vi "Dashboard Main.vi"() -> ()   [LabVIEW 2016]
uses:
  <vilib>/Utility/miscctls.llb/LVRowAndColumnTypeDef.ctl
  <vilib>/event_ctls.llb/eventvkey.ctl
  <vilib>/Rock Robotics/Network Tables/NT Read Numeric Array.vi
  <vilib>/Rock Robotics/Network Tables/NT Write Boolean.vi
  <vilib>/Rock Robotics/Network Tables/NT Read Boolean.vi
  <vilib>/Rock Robotics/WPI/Dashboard/WPI_DashboardLogging Global.vi
panel:
  in  "Camera Settings Right":T1={"Frame Rate"=30, "Compression"=30, "Size"=1, "DB Camera Config"=FALSE} {"Frame Rate" scale=1.0..30.0; "Compression" scale=100.0..-1.0; "Size" items=["640x480", "320x240", "160x120"]}
  in  "Camera Name Right":string(combo)="No Camera Selection"
  out "Camera Info":cluster{"Mbps LED":bool, "Mbps":dbl, "fps":dbl} {"fps" format="%#.1g"; "Mbps" format="%#.1g"}
  in  "Camera Settings":T1={"Frame Rate"=30, "Compression"=30, "Size"=1, "DB Camera Config"=FALSE} {"Frame Rate" scale=1.0..30.0; "Compression" scale=100.0..-1.0; "Size" items=["640x480", "320x240", "160x120"]}
  in  "TCP":refnum<k5>
  in  "Rec Mode":enum32{"Stop", "Record", "Playback"}(radio)
  out "Robot IP":string
  out "Image Message":string="Timeout in Camera Communications"
  in  "Dashboard Tab":T2(tab)
  out "Auto Aim":bool
  out "Vision Degrees":dbl
  out "Distance":dbl
  out "Score":dbl
  out "Shooter":bool
  in  "Compressor":bool
  in  "Delay":dbl(slide) scale=0.0..10.0
  out "RPM":dbl(knob) scale=0.0..10.0
  out "Right":dbl
  out "Left":dbl
  in  "Select Auto":string(combo)="Select Autonomous ..."
  out "NT Connection":bool
  out "MotorChart R":cluster{"Numeric":dbl, "Numeric":dbl}(graph)
  out "MotorChart L":cluster{"Numeric":dbl, "Numeric":dbl}(graph)
  out "MotorSliders R":cluster{"MotorSlide1":dbl, "MotorSlide2":dbl} {"MotorSlide2" scale=-1.0..1.0 scale format="%#_2e"; "MotorSlide1" scale=-1.0..1.0 scale format="%#_2e"}
  out "MotorSliders L":cluster{"MotorSlide1":dbl, "MotorSlide2":dbl} {"MotorSlide2" scale=-1.0..1.0 scale format="%#_2e"; "MotorSlide1" scale=-1.0..1.0 scale format="%#_2e"}
  out "Gyro":dbl(knob) scale=0.0..360.0
  out "JS1 Z":dbl(slide) scale=-1.0..1.0 scale format="%#_2e"
  out "JS1 Graph":cluster{"X":dbl, "Y":dbl}[](graph)
  out "JS1 Buttons":T3
  out "JS2 Z":dbl(slide) scale=-1.0..1.0 scale format="%#_2e"
  out "JS2 Graph":cluster{"X":dbl, "Y":dbl}[](graph)
  out "JS2 Buttons":T3
  out "Mode":T4(ring)=enum."Auto Disabled"
  out "Camera Image Right":T5(plugin-control)
  in  "DB/String 9":string
  in  "DB/String 8":string
  in  "DB/String 7":string
  in  "DB/String 6":string
  in  "DB/String 5":string
  in  "DB/String 4":string
  in  "DB/String 3":string
  in  "DB/String 2":string
  in  "DB/String 1":string
  in  "DB/String 0":string
  in  "DB/Slider 0":dbl(slide) scale=0.0..5.0
  in  "DB/Slider 1":dbl(slide) scale=0.0..5.0
  in  "DB/Slider 2":dbl(slide) scale=0.0..5.0
  in  "DB/Slider 3":dbl(slide) scale=0.0..5.0
  out "DB/LED 3":bool
  out "DB/LED 2":bool
  out "DB/LED 1":bool
  out "DB/LED 0":bool
  in  "DB/Button 3":bool
  in  "DB/Button 2":bool
  in  "DB/Button 1":bool
  in  "DB/Button 0":bool caption="New Name"
  in  "Test Slider":dbl(slide) scale=0.0..100.0 scale format="%#_3g"
  in  "On/Off":bool caption="Solenoid"
  in  "Test Name":u16(ring) items=["Select the test to run..."]
  in  "Test Tree":string(tree)
  in  "Motor":cluster{"Value":dbl, "Enable":bool} {"Value" scale=-1.0..1.0 scale format="%#_3g"}
  out "Progress":T6 {"Test Progress" scale=0.0..100.0}
  in  "Rev/Fwd":cluster{"Forward":bool, "Reverse":bool}
  in  "Test Ring":u16(ring) items=["Monochrome", "Color"]
  out "Cmd Status":string
  in  "Execute Command":bool
  in  "Command Params":string[][](table)
  in  "Command Selection":i32(listbox)
  in  "CheckList":i32(listbox)
  out "Tree":string(tree)
  out "Camera Image":T5(plugin-control)
  out "Background":bool
  in  "Camera Name":string(combo)="No Camera Selection"
  # "HW"
  # "HW"
  # "Joysticks"
  # "Drive Motors"
  # "Front"
  # "Right"
  # "Left"
  # "Back"
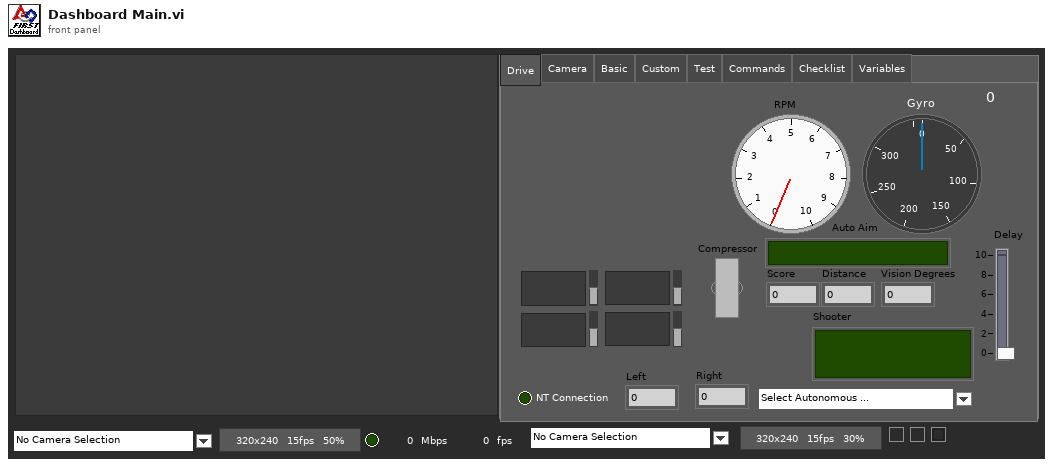
[diagram p1: front panel]
types:
  T1 = cluster{"Frame Rate":i32, "Compression":i32, "Size":u16, "DB Camera Config":bool}
  T2 = enum32{"Drive", "Camera", "Basic", "Custom", "Test", "Commands", "Checklist", "Variables"}
  T3 = cluster{bool, bool, bool, bool, bool, bool, bool, bool, bool, bool, bool, bool}
  T4 = enum8{"Tele-Op Disabled", "Tele-Op Enabled", "Auto Disabled", "Auto Enabled", "Test Disabled", "Test Enabled", "Disconnected", "No Code", "E-Stop"}
  T5 = typedef "IMAQ Image.ctl" = refnum<image>
  T6 = cluster{"Test Progress":u8, "Test Progress Text":string}
  T7 = typedef "Image Type" = u32
  T8 = cluster{"IDs":cluster{"RPC field ID":u16, "Unique ID":u16}, "String":string}
  T9 = enum32{"Drive", "Basic", "Custom", "Test", "Checklist", "Variables"}
  T10 = cluster{"Error Strings":string, "Disable Counts":cluster{u16, u16}, "Rail Faults":cluster{u16, u16, u16}, "Robot IP":string, "DB Mode":u8, "Event Info":cluster{"Name":string, "Type":u8, "Number":u16, "Replay":u8}}
  T11 = cluster{"Storage":cluster{"Disk Free":u64, "RAM Block":u32, "RAM free":u32}, "CPU Utilization":cluster{"CPU % ISR":sgl, "CPU % Time Crit":sgl, "CPU % Timed Str":sgl, "CPU % High":sgl, "CPU % Above":sgl, "CPU % Normal":sgl, "CPU % Low":sgl}, "CAN":cluster{"% Bus Utilization":sgl, "Bus Off Cnt":u32, "TX_FIFO Full Cnt":u32, "Receive Error Cnt":u8, "Transmit Error Cnt":u8}, "HID":cluster{"HID Outputs":u32, "Rumble Low":u16, "Rumble High":u16}[]}
  T12 = cluster{"Status bits":cluster{"Test Mode":bool, "Autonomous":bool, "Enabled":bool, "Code Start":bool, "Brownout":bool, "Reserved 2":bool, "Reserved 3":bool, "E-Stop":bool}, "Code Trace":cluster{"Disabled":bool, "TeleOp":bool, "Auto":bool, "Test":bool}, "Controller Type":enum16{"unknown", "cRIO", "roboRio"}, "Code?":enum16{"unknown", "noCode", "code"}, "Battery V":dbl}
  T13 = cluster{"Control Bits":cluster{"TestMode":bool, "Autonomous":bool, "Enabled":bool, "FMS Present":bool, bool, bool, bool, "E-Stop":bool}, "Team Station ":u8, "Countdown":sgl, "Joystick Values":cluster{"Axes":dbl[], "Buttons":bool[], "POVs":i16[]}[]}
  T14 = cluster{"Axes":dbl[], "Buttons":bool[], "POVs":i16[]}[]
  T15 = cluster{"Axes":dbl[], "Buttons":bool[], "POVs":i16[]}
  T16 = cluster{"Buttons[0]":bool, "Buttons[1]":bool, "Buttons[2]":bool, "Buttons[3]":bool, "Buttons[4]":bool, "Buttons[5]":bool, "Buttons[6]":bool, "Buttons[7]":bool, "Buttons[8]":bool, "Buttons[9]":bool, "Buttons[10]":bool, "Buttons[11]":bool}
  T17 = cluster{"Camera Image":refnum<vi>, "Dashboard Tab":refnum<vi>, "Background":refnum<vi>, "Rec Mode":refnum<vi>, "Test Slider":refnum<vi>, "On/Off ":refnum<vi>, "Test Ring":refnum<vi>, "Rev/Fwd":refnum<vi>, "Test Name":refnum<vi>, "Motor":refnum<vi>, "Progress":refnum<vi>, "CheckList":refnum<vi>, "Tree":refnum<vi>, "Test Tree":refnum<vi>, "Command Params":refnum<vi>, "Command Selection":refnum<vi>, "Execute Command":refnum<vi>, "Cmd Status":refnum<vi>, "Camera Settings":refnum<vi>, "Camera Name":refnum<vi>, "Camera Info":refnum<vi>, "Camera Settings Right":refnum<vi>, "Camera Name Right":refnum<vi>, "Camera Image Right":refnum<vi>}
  T18 = cluster{"Operation":enum16{"Update", "Clear"}, "Color Box":u32}[]
  T19 = typedef "eventvkey.ctl" = enum16{"ASCII", "Enter", "Return", "Shift", "Ctrl", "Alt", "Cmd", "Opt", "Caps", "NumLock", "Clear", "Break", "Up", "Down", "Left", "Right", "Insert", "Delete", "Home", "End", "PageUp", "PageDown", "Escape", "Help", "Pause", "ScrollLock", "F1", "F2", "F3", "F4", "F5", "F6", "F7", "F8", "F9", "F10", "F11", "F12", "F13", "F14", "F15", "F16", "F17", "F18", "F19", "F20", "F21", "F22", "F23", "F24", "Play", "VolumeUp", "VolumeDown", "Mute", "Two Byte Char"}
  T20 = cluster{"Image Size":bool, "Image Type":bool, "Pixel Value":bool, "ROI Information":bool, "Zoom Factor":bool}
  T21 = cluster{"Operation":enum16{"Update", "Clear"}, "Color Box":u32}
  T22 = typedef "LVRowAndColumnTypeDef.ctl" = cluster{"Row":i32, "Column":i32}
  T23 = cluster{"Shift":bool, "Ctrl":bool, "Alt":bool, "Cmd":bool, "Opt":bool}
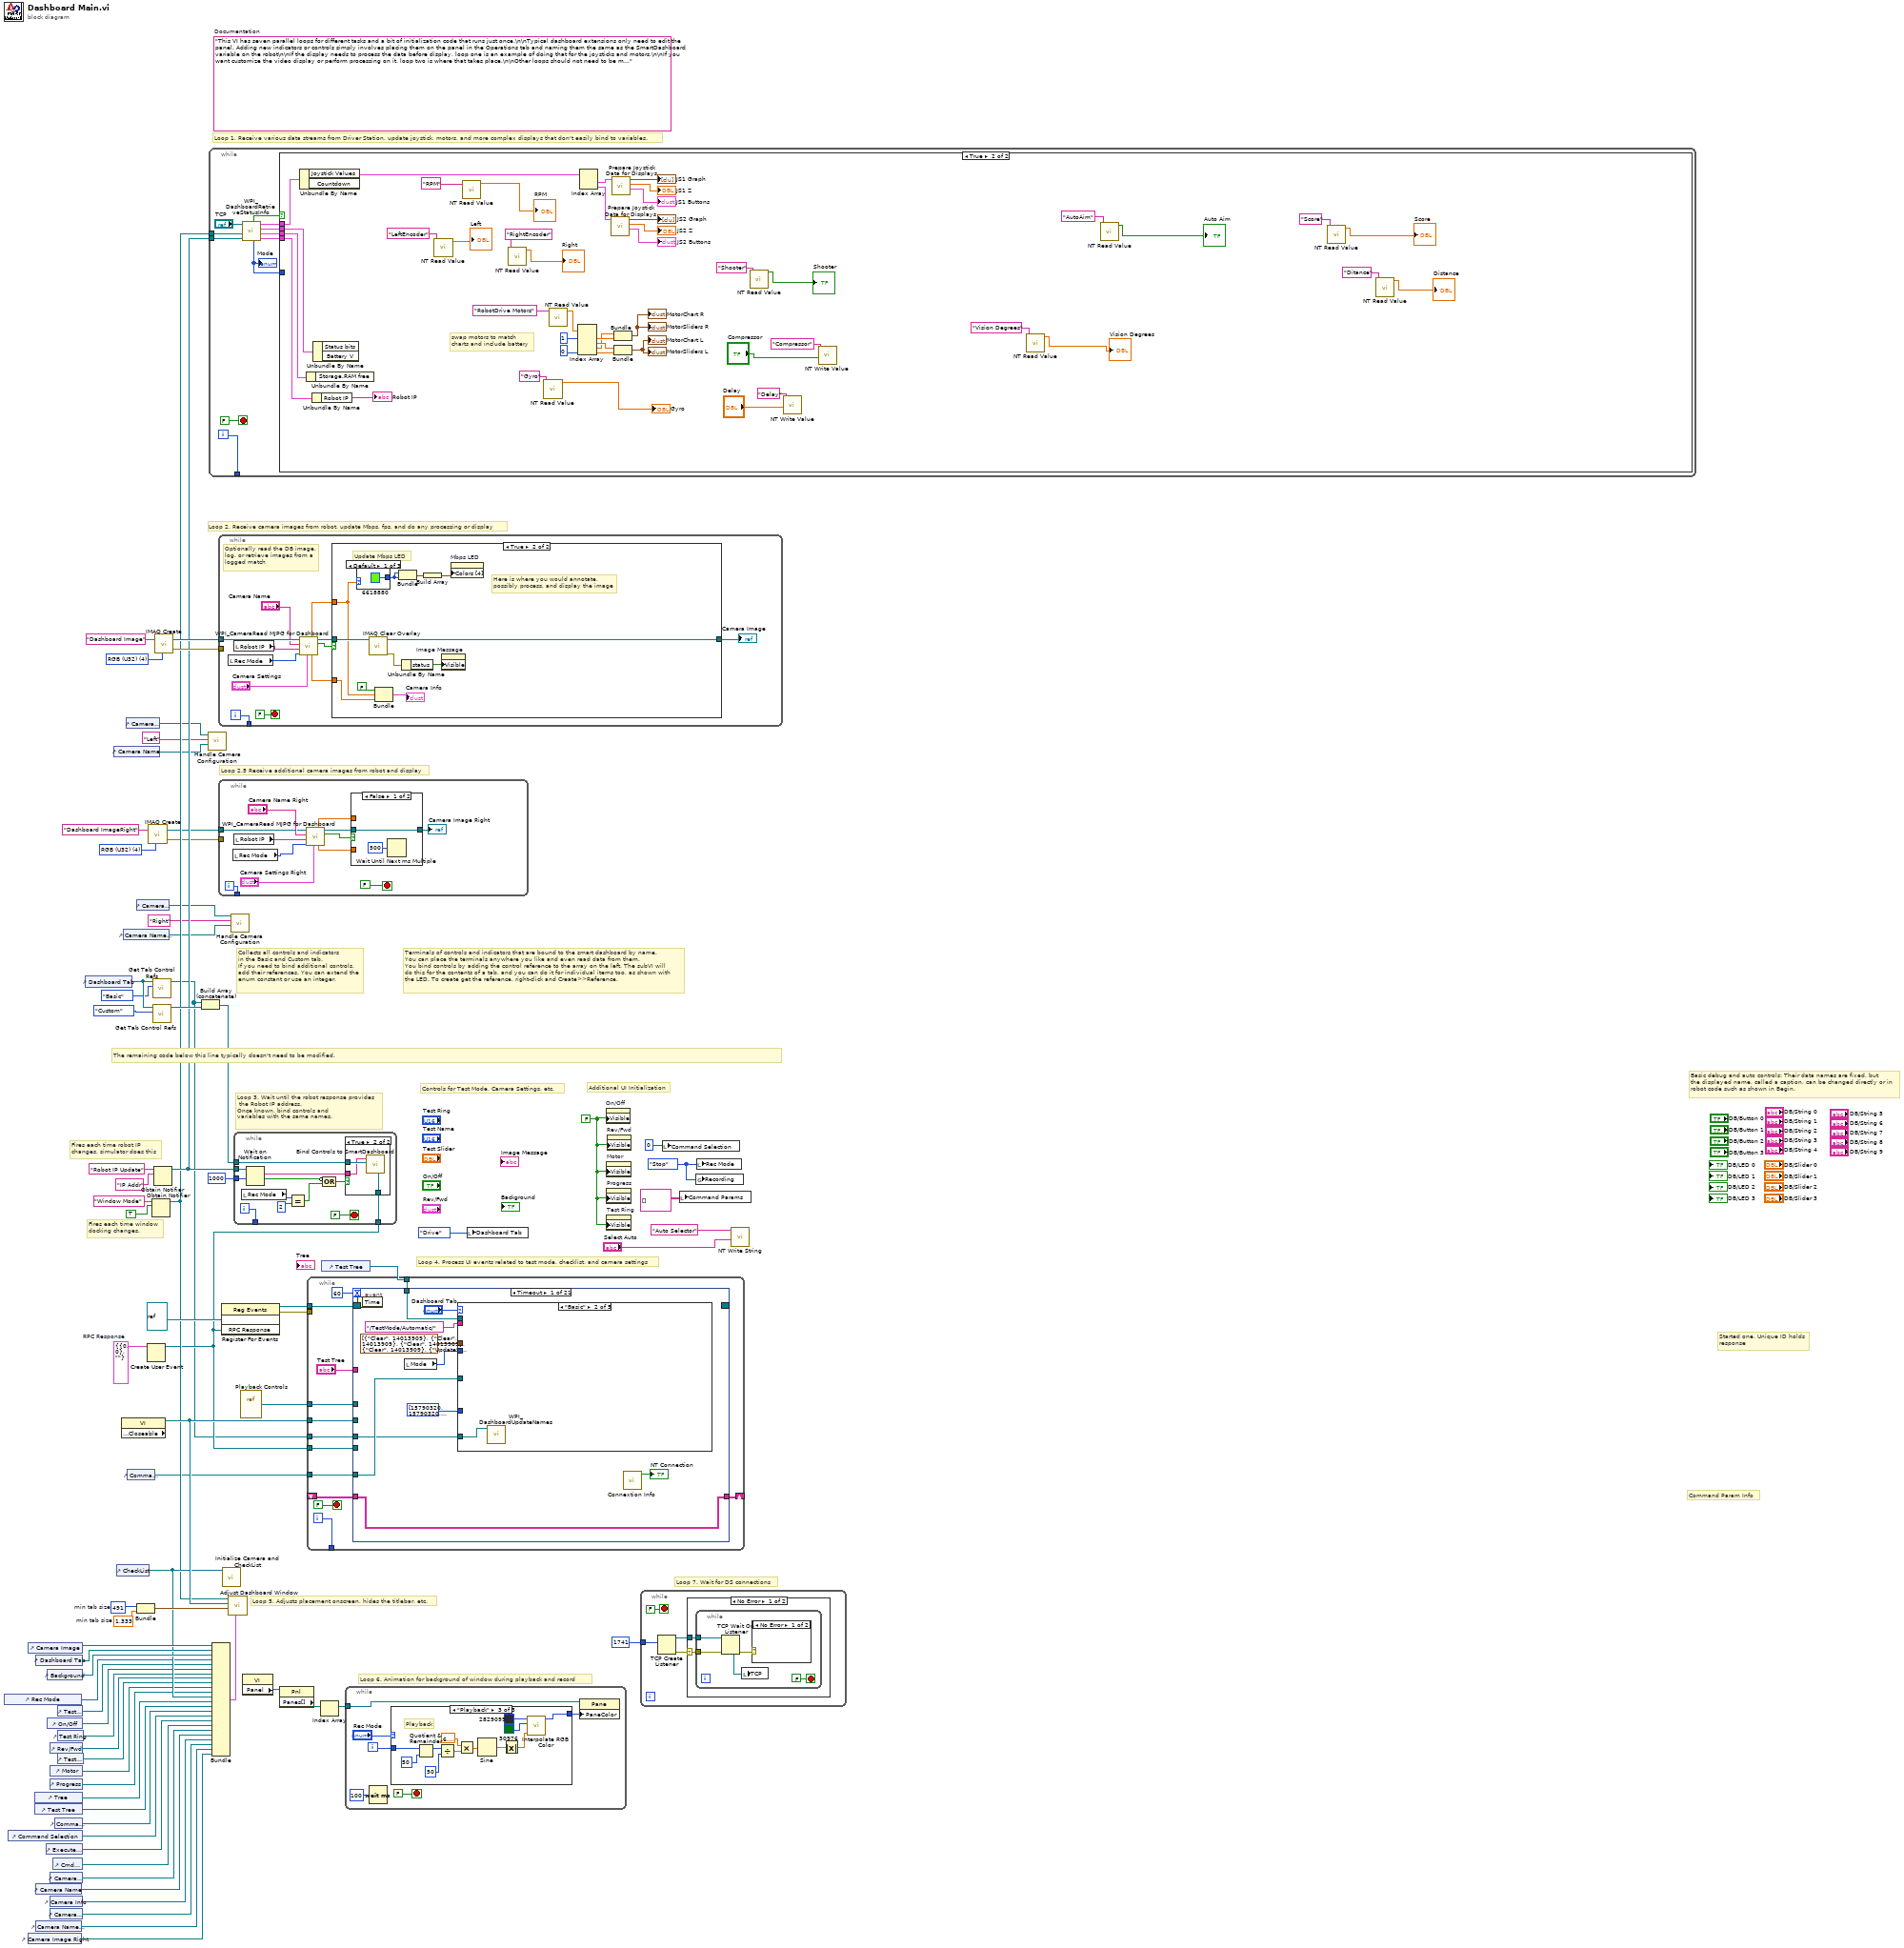
[diagram p0: block diagram]
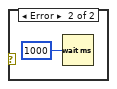
[diagram p3: hidden frame]
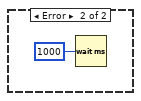
[diagram p4: hidden frame]
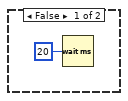
[diagram p5: hidden frame]
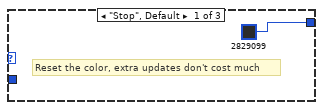
[diagram p6: hidden frame]
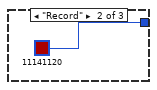
[diagram p7: hidden frame]
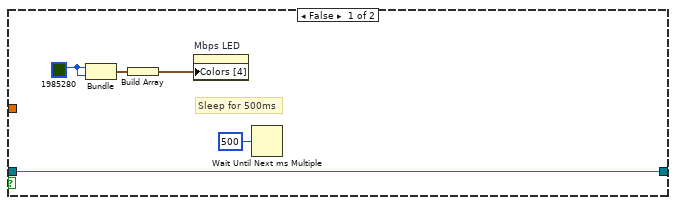
[diagram p9: hidden frame]
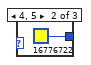
[diagram p10: hidden frame]
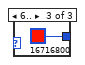
[diagram p11: hidden frame]
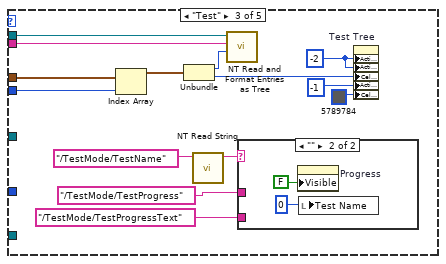
[diagram p13: hidden frame]
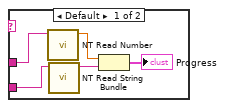
[diagram p14: hidden frame]
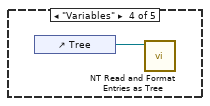
[diagram p15: hidden frame]
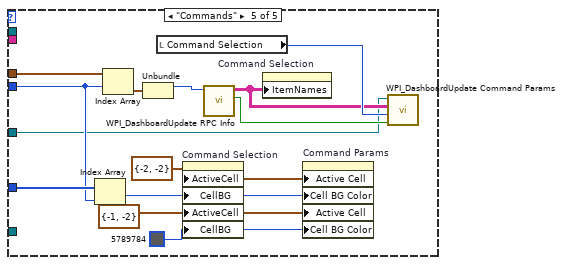
[diagram p16: hidden frame]
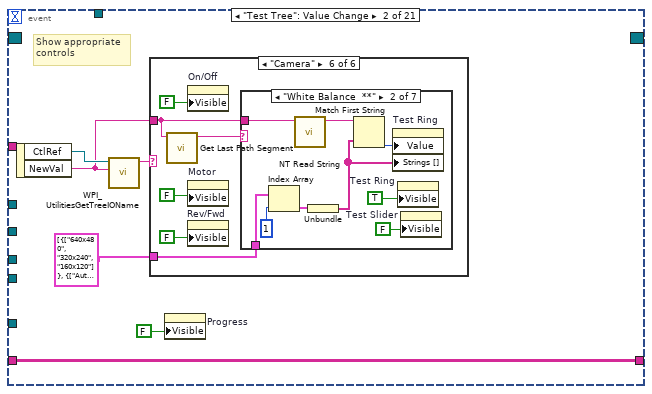
[diagram p17: hidden frame]
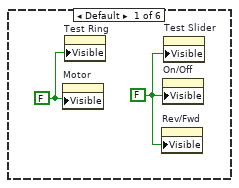
[diagram p18: hidden frame]
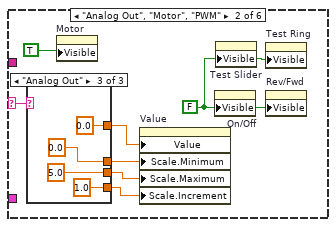
[diagram p19: hidden frame]
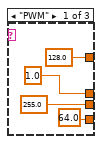
[diagram p20: hidden frame]
diagram:
  w10 = T7 4 items=["Grayscale (U8)", "Grayscale (I16)", "Grayscale (SGL)", "Complex (CSG)", "RGB (U32)", "HSL (U32)", "RGB (U64)"] ("Image Type")
  w26 = T8 {"IDs"={"RPC field ID"=0, "Unique ID"=0}, "String"=""}  # RPC Response
  w51 = 491  # min tab size
  w50 = 1.333  # min tab size
  w58 = enum32{"Stop", "Record", "Playback"}."Stop" ("Rec Mode")
  w33 = FALSE ("Visible")
  (unwired) "This VI has seven parallel loops for different tasks and a bit of initialization code that runs just once.\n\nTypical dashboard extensions only need to edit the panel. Adding new indicators or controls simply involves placing them on the panel in the Operations tab and naming them the same as the SmartDashboard variable on the robot\n\nIf the display needs to process the data before display, loop one is an example of doing that for the joysticks and motors.\n\nIf you want customize the video display or perform processing on it, loop two is where that takes place.\n\nOther loops should not need to be modified. They are pretty standard, and document the task they perform."  # Documentation
  w75 = T7 4 items=["Grayscale (U8)", "Grayscale (I16)", "Grayscale (SGL)", "Complex (CSG)", "RGB (U32)", "HSL (U32)", "RGB (U64)"] ("Image Type")
  # "Loop 2.5 Receive additional camera images from robot and display"
  # "Command Param Info"
  # "Started one, Unique ID holds\nresponse"
  # "Loop 7. Wait for DS connections"
  # "Basic debug and auto controls: Their data names are fixed, but\nthe displayed name, called a caption, can be changed directly or in\nrobot code such as shown in Begin."
  # "Controls for Test Mode, Camera Settings, etc."
  # "Additional UI Initialization"
  # "Loop 6. Animation for background of window during playback and record"
  # "Fires each time robot IP\nchanges, simulator does this"
  # "Fires each time window\ndocking changes."
  # "Collects all controls and indicators\nin the Basic and Custom tab.\nIf you need to bind additional controls,\nadd their references. You can extend the\nenum constant or use an integer."
  # "The remaining code below this line typically doesn't need to be modified."
  # "Loop 4. Process UI events related to test mode, checklist, and camera settings"
  # "Terminals of controls and indicators that are bound to the smart dashboard by name.\nYou can place the terminals anywhere you like and even read data from them.\nYou bind controls by adding the control reference to the array on the left. The subVI will\ndo this for the contents of a tab, and you can do it for individual items too, as shown with\nthe LED. To create get the reference, right-click and Create>>Reference."
  # "Loop 3. Wait until the robot response provides\n the Robot IP address.\nOnce known, bind controls and\nvariables with the same names."
  # "Loop 5. Adjusts placement onscreen, hides the titlebar, etc."
  # "Loop 1. Receive various data streams from Driver Station, update joystick, motors, and more complex displays that don't easily bind to variables."
  # "Loop 2. Receive camera images from robot, update Mbps, fps, and do any processing or display"
  n1 = control-ref of="Rec Mode"() -> (w39:refnum<vi>)
  n2 = control-ref of="Command Selection"() -> (w25:refnum<vi>)
  n3 = control-ref of="Camera Image Right"() -> (w1:refnum<vi>)
  n4 = control-ref of="Camera Image"() -> (w53:refnum<vi>)
  n5 = control-ref of="Tree"() -> (w43:refnum<vi>)
  n6 = control-ref of="Test Tree"() -> (w42:refnum<vi>)
  n7 = control-ref of="Dashboard Tab"() -> (w52:refnum<vi>)
  n8 = control-ref of="Camera Name"() -> (w16:refnum<vi>)
  n9 = control-ref of="Camera Name Right"() -> (w2:refnum<vi>)
  n10 = control-ref of="Execute Command"() -> (w27:refnum<vi>)
  n11 = control-ref of="Background"() -> (w48:refnum<vi>)
  n12 = control-ref of="On/Off"() -> (w37:refnum<vi>)
  n13 = control-ref of="Progress"() -> (w34:refnum<vi>)
  n14 = control-ref of="Camera Settings"() -> (w17:refnum<vi>)
  n15 = control-ref of="Camera Info"() -> (w15:refnum<vi>)
  n16 = control-ref of="Camera Settings Right"() -> (w3:refnum<vi>)
  n17 = control-ref of="Rev/Fwd"() -> (w35:refnum<vi>)
  n18 = control-ref of="Motor"() -> (w40:refnum<vi>)
  n19 = control-ref of="Cmd Status"() -> (w21:refnum<vi>)
  n20 = control-ref of="Command Params"() -> (w28:refnum<vi>)
  n21 = control-ref of="Test Slider"() -> (w38:refnum<vi>)
  n22 = control-ref of="Test Ring"() -> (w36:refnum<vi>)
  n23 = control-ref of="Test Name"() -> (w41:refnum<vi>)
  n24 = control-ref of="Dashboard Tab"() -> (w56:refnum<vi>)
  n25 = control-ref of="Camera Name"() -> (w18:refnum<vi>)
  n26 = control-ref of="CheckList"() -> (w44:refnum<vi>)
  n27 = property class="VI" props=["Front Panel.Closeable"]() -> (reference out=w57:refnum<vi>)  [unwired: 2 in, 2 out]
  n28 = control-ref of="Camera Name Right"() -> (w6:refnum<vi>)
  n29 = control-ref of="Camera Settings"() -> (w19:refnum<vi>)
  n30 = control-ref of="Command Params"() -> (w20:refnum<vi>)
  n31 = control-ref of="Camera Settings Right"() -> (w7:refnum<vi>)
  n32 = Bundle("min tab size"=w51, "min tab size"=w50) -> (w49:cluster{"min tab size":i32, "min tab size":dbl})  [unwired: 1 in]
  n33 = Create User Event(user event datatype=w26) -> (user event=w22:refnum<user-event>)  [unwired: 1 in, 1 out]
  n34 = call "IMAQ Create"("Image Name"="Dashboard ImageRight", "Image Type"=w10) -> ("New Image"=w9:T5, "error out"=w8:errorcluster)  [unwired: 2 in, 1 out]
  n35 = Obtain Notifier(name (unnamed)="Window Mode", notification data type=TRUE) -> (notifier out=w31:refnum<notifier>)  [unwired: 2 in, 2 out]
  n36 = call <vilib>:"Get Tab Control Refs.vi"("Page Index"=T9."Basic" ("Dashboard Tab"), "TabControl in"=w56) -> ("ControlsOnPage"=w14:refnum<vi>[])  [unwired: 9 in]
  n37 = call <vilib>:"Get Tab Control Refs.vi"("Page Index"=T9."Custom" ("Dashboard Tab"), "TabControl in"=w56) -> ("ControlsOnPage"=w55:refnum<vi>[])  [unwired: 9 in]
  n38 = Obtain Notifier(name (unnamed)="Robot IP Update", notification data type="IP Addr" ("name (unnamed)")) -> (notifier out=w32:refnum<notifier>)  [unwired: 2 in, 2 out]
  n39 = call "IMAQ Create"("Image Name"="Dashboard Image", "Image Type"=w75) -> ("New Image"=w73:T5, "error out"=w72:errorcluster)  [unwired: 2 in, 1 out]
  n40 = Build Array (concatenate)(w14, w55) -> (w54:refnum<vi>[])
  n41 = call "Handle Camera Configuration.vi"("CameraNameRef"=w18, "Camera File Name"="Left", "ClusterRef"=w19) -> ()  [unwired: 9 in]
  n42 = while {
    tunnel: [w85] -> _
    tunnel: w32 -> [w79]
    tunnel: w31 -> [w76]
    i -> [w85]
    stop <- FALSE stop-if-true
    n43 = call <vilib>:"WPI_DashboardRetrieveStatusInfo.vi"("Binding Refnum"=w79, "Window Mode Notifier"=w76, "TCP Cnx"="TCP") -> ("Power and Errors"=w80:T10, "Robot Metrics"=w83:T11, "Status Info"=w84:T12, "Control Info"=w81:T13, "Robot Mode"=w78:T4, "Process?"=w82:bool)  [unwired: 3 in]
    "Mode" <- w78
    n44 = case shown="True" w82 {
      tunnel: w84 -> [_ w133]
      tunnel: w83 -> [_ w132]
      tunnel: w81 -> [_ w131]
      tunnel: w80 -> [_ w130]
      tunnel: w78 -> [_ _]
      frame False {
        n45 = Wait (ms)(milliseconds to wait=u32 20) -> ()  [unwired: 1 out]
      }
      frame True {
        # "swap motors to match\ncharts and include battery"
        n46 = Unbundle By Name(w131) -> ("Joystick Values"=w121:T14)  [unwired: 1 out]
        n47 = Unbundle By Name(w132) -> ()  [unwired: 1 out]
        n48 = Unbundle By Name(w130) -> ("Robot IP"=→"Robot IP":string)
        n49 = Unbundle By Name(w133) -> ()  [unwired: 2 out]
        n50 = call-poly <vilib>:"NT Read Value.vi"("Name"="LeftEncoder") -> ("Numeric"=→"Left":dbl)  [unwired: 9 in, 1 out]
        n51 = call-poly <vilib>:"NT Read Value.vi"("Name"="RPM") -> ("Numeric"=→"RPM":dbl)  [unwired: 9 in, 1 out]
        n52 = call-poly <vilib>:"NT Read Value.vi"("Name"="RightEncoder") -> ("Numeric"=→"Right":dbl)  [unwired: 9 in, 1 out]
        n53 = call-poly <vilib>:"NT Read Value.vi"("Name"="Gyro") -> ("Numeric"=→"Gyro":dbl)  [unwired: 9 in, 1 out]
        n54 = call-poly <vilib>:"NT Read Value.vi"("Name"="RobotDrive Motors") -> ("Numeric Array"=w111:dbl[])  [unwired: 9 in, 1 out]
        n55 = Index Array(array=w111, index #1=1, index #4=0) -> (element #1=w125:dbl, element #2=w126:dbl, element #3=w124:dbl, element #4=w129:dbl)  [unwired: 2 in]
        n56 = Index Array(array=w121) -> (element #1=w120:T15, element #2=w116:T15)  [unwired: 2 in]
        n57 = call "Prepare Joystick Data for Displays.vi"("Joystick Values"=w116) -> ("Buttons"=→"JS2 Buttons":T16, "Z Axis"=→"JS2 Z":dbl, "Cartesian Data"=→"JS2 Graph":cluster{"X axis":dbl, "X axis":dbl}[])  [unwired: 8 in]
        n58 = call "Prepare Joystick Data for Displays.vi"("Joystick Values"=w120) -> ("Buttons"=→"JS1 Buttons":T16, "Z Axis"=→"JS1 Z":dbl, "Cartesian Data"=→"JS1 Graph":cluster{"X axis":dbl, "X axis":dbl}[])  [unwired: 8 in]
        n59 = Bundle("Numeric"=w124, "Numeric"=w125) -> (→"MotorChart R" →"MotorSliders R":cluster{"Numeric":dbl, "Numeric":dbl})  [unwired: 1 in]
        n60 = Bundle("Numeric"=w126, "Numeric"=w129) -> (→"MotorChart L" →"MotorSliders L":cluster{"Numeric":dbl, "Numeric":dbl})  [unwired: 1 in]
        n61 = call-poly <vilib>:"NT Read Value.vi"("Name"="Shooter") -> ("Boolean"=→"Shooter":bool)  [unwired: 9 in, 1 out]
        n62 = call-poly <vilib>:"NT Write Value.vi"("Numeric"="Delay", "Name"="Delay") -> ()  [unwired: 9 in, 1 out]
        n63 = call-poly <vilib>:"NT Write Value.vi"("Boolean"="Compressor", "Name"="Compressor") -> ()  [unwired: 9 in, 1 out]
        n64 = call-poly <vilib>:"NT Read Value.vi"("Name"="Vision Degrees") -> ("Numeric"=→"Vision Degrees":dbl)  [unwired: 9 in, 1 out]
        n65 = call-poly <vilib>:"NT Read Value.vi"("Name"="AutoAim") -> ("Boolean"=→"Auto Aim":bool)  [unwired: 9 in, 1 out]
        n66 = call-poly <vilib>:"NT Read Value.vi"("Name"="Score") -> ("Numeric"=→"Score":dbl)  [unwired: 9 in, 1 out]
        n67 = call-poly <vilib>:"NT Read Value.vi"("Name"="Ditance") -> ("Numeric"=→"Distance":dbl)  [unwired: 9 in, 1 out]
      }
    }
  }
  n68 = Bundle("Camera Image"=w53, "Dashboard Tab"=w52, "Background"=w48, "Rec Mode"=w39, "Test Slider"=w38, "On/Off"=w37, "Test Ring"=w36, "Rev/Fwd"=w35, "Test Name"=w41, "Motor"=w40, "Progress"=w34, "CheckList"=w44, "Tree"=w43, "Test Tree"=w42, "Command Params"=w28, "Command Selection"=w25, "Execute Command"=w27, "Cmd Status"=w21, "Camera Settings"=w17, "Camera Name"=w16, "Camera Info"=w15, "Camera Settings Right"=w3, "Camera Name Right"=w2, "Camera Image Right"=w1) -> (w45:T17)  [unwired: 1 in]
  n69 = while {
    tunnel: w73 -> [w143]
    tunnel: w72 -> [_]
    tunnel: [w144] -> _
    i -> [w144]
    stop <- FALSE stop-if-true
    # "Optionally read the DB image,\nlog, or retrieve images from a\nlogged match"
    n70 = local read "Rec Mode"() -> (w139:enum32{"Stop", "Record", "Playback"})
    n71 = local read "Robot IP"() -> (w138:string)
    n72 = call <vilib>:"WPI_CameraRead MJPG for Dashboard.vi"("Camera Settings"="Camera Settings", "Rec Mode"=w139, "Robot IP"=w138, "Camera Name"="Camera Name", "Refnum in"=w143) -> ("Active"=w141:bool, "Refnum out"=w142:T5, "FPS"=w140:dbl, "Bandwidth (Mbps)"=w137:dbl)  [unwired: 3 in]
    n73 = case shown="True" w141 {
      tunnel: w142 -> [w146 w157]
      tunnel: w137 -> [_ w154]
      tunnel: w140 -> [_ w155]
      tunnel: [w146 w151] -> w134
      frame False {
        w148 = u32 1985280 ("Color Box")
        # "Sleep for 500ms"
        n74 = Bundle("Color Box"=w148, "Color Box"=w148) -> (w149:cluster{"Color Box":u32, "Color Box":u32})  [unwired: 1 out]
        n75 = Build Array(w149) -> (w147:cluster{"Color Box":u32, "Color Box":u32}[])
        n76 = property on="Mbps LED" class="Bool (strict)"("Colors [4]"=w147) -> ()  [unwired: 2 in, 2 out]
        n77 = Wait Until Next ms Multiple(millisecond multiple=u32 500) -> ()  [unwired: 1 out]
      }
      frame True {
        # "Here is where you would annotate,\npossibly process, and display the image"
        # "Update Mbps LED"
        n78 = case shown="Default" w154 {
          tunnel: [u32 6618880 ("Color Box") u32 16776722 ("Color Box") u32 16716800 ("Color Box")] -> w158
          frame Default {
          }
          frame 4, 5 {
          }
          frame 6.. {
          }
        }
        n79 = call "IMAQ Clear Overlay"("Image"=w157) -> ("error out"=w160:errorcluster, "Image Out"=w151:T5)  [unwired: 2 in, 7 out]
        n80 = Bundle(FALSE, "Bandwidth (Mbps)"=w154, "FPS"=w155) -> (→"Camera Info":cluster{bool, "Bandwidth (Mbps)":dbl, "FPS":dbl})  [unwired: 1 in]
        n81 = Bundle("Color Box"=w158, "Color Box"=w158) -> (w159:cluster{"Color Box":u32, "Color Box":u32})  [unwired: 1 out]
        n82 = Unbundle By Name(w160) -> ("status"=w161:bool)
        n83 = Build Array(w159) -> (w156:cluster{"Color Box":u32, "Color Box":u32}[])
        n84 = property on="Image Message" class="Str"("Visible"=w161) -> ()  [unwired: 2 in, 2 out]
        n85 = property on="Mbps LED" class="Bool (strict)"("Colors [4]"=w156) -> ()  [unwired: 2 in, 2 out]
      }
    }
    "Camera Image" <- w134
  }
  n86 = while {
    tunnel: w9 -> [w175]
    tunnel: w8 -> [_]
    tunnel: [w169] -> _
    i -> [w169]
    stop <- FALSE stop-if-true
    n87 = local read "Rec Mode"() -> (w173:enum32{"Stop", "Record", "Playback"})
    n88 = local read "Robot IP"() -> (w174:string)
    n89 = call <vilib>:"WPI_CameraRead MJPG for Dashboard.vi"("Camera Settings"="Camera Settings Right", "Rec Mode"=w173, "Robot IP"=w174, "Camera Name"="Camera Name Right", "Refnum in"=w175) -> ("Active"=w168:bool, "Refnum out"=w171:T5, "FPS"=w166:dbl, "Bandwidth (Mbps)"=w167:dbl)  [unwired: 3 in]
    n90 = case shown="False" w168 {
      tunnel: w171 -> [w177 w179]
      tunnel: w167 -> [_ _]
      tunnel: w166 -> [_ _]
      tunnel: [w177 w179] -> w165
      frame False {
        n91 = Wait Until Next ms Multiple(millisecond multiple=u32 500) -> ()  [unwired: 1 out]
      }
      frame True {
      }
    }
    "Camera Image Right" <- w165
  }
  n92 = register-events(refnum<vi> refnum, w22) -> (reference out=w62:refnum<event-registration>, error out=w61:errorcluster)  [unwired: 2 in]
  n93 = call "Initialize Camera and CheckList.vi"("ListBox in"=w44) -> ()  [unwired: 11 in]
  n94 = call "Adjust Dashboard Window.vi"("Sizing Refnums"=w45, "Size Constraints"=w49, "VI"=w57, "WIn Mode"=w31) -> ()  [unwired: 8 in]
  n95 = call "Handle Camera Configuration.vi"("CameraNameRef"=w6, "Camera File Name"="Right", "ClusterRef"=w7) -> ()  [unwired: 9 in]
  n96 = while {
    tunnel: w54 -> [w191]
    tunnel: w32 -> [w189]
    tunnel: [w187] -> _
    tunnel: u32 1000 ("milliseconds to wait") -> [w186]
    tunnel: w22 -> [w180]
    i -> [w187]
    stop <- FALSE stop-if-true
    n97 = local read "Rec Mode"() -> (w182:enum32{"Stop", "Record", "Playback"})
    n98 = Wait on Notification(notifier=w189, timeout in ms (-1)=w186) -> (notification=w188:string, timed out?=w184:bool)  [unwired: 2 in, 2 out]
    n99 = Equal?(x=w182, y=u16 2 ("Rec Mode")) -> (x = y?=w183:bool)
    n100 = Compound Arithmetic op=OR(invert w184, w183) -> (w185:bool)
    n101 = case shown="True" w185 {
      tunnel: w191 -> [_ w194]
      tunnel: w188 -> [_ w193]
      tunnel: w180 -> [_ w192]
      frame False {
      }
      frame True {
        n102 = call <vilib>:"Bind Controls to SmartDashboard.vi"("RPC ref"=w192, "Bound Control Refs"=w194, "Server IP Address"=w193) -> ()  [unwired: 9 in]
      }
    }
  }
  n103 = vi-ref "Playback Controls.vi"() -> (w63:refnum<vi>)
  n104 = property class="VI"() -> ("Panel"=w65:refnum<vi>)  [unwired: 2 in, 2 out]
  n105 = property class="Pnl"(reference=w65) -> ("Panes[]"=w66:refnum<vi>[])  [unwired: 1 in, 2 out]
  n106 = Index Array(array=w66) -> (element=w64:refnum<vi>)  [unwired: 1 in]
  n107 = control-ref of="Test Tree"() -> (w67:refnum<vi>)
  n108 = while {
    tunnel: [w204] -> _
    tunnel: w67 -> [w203]
    tunnel: w63 -> [w202]
    tunnel: w62 -> [w201]
    tunnel: w61 -> [_]
    tunnel: w57 -> [w200]
    tunnel: w22 -> [w199]
    tunnel: w20 -> [w198]
    shift-right: [w197] -> _
    shift-left: _ -> [w196]
    tunnel: w14 -> [w195]
    i -> [w204]
    stop <- FALSE stop-if-true
    n109 = event shown="[0] Timeout" {
      selector: w201 -> [_ _ _ _ _ _ _ _ _ _ _ _ _ _ _ _ _ _ _ _ _]
      dyn-events: [_ _ _ _ _ _ _ _ _ _ _ _ _ _ _ _ w460 _ _ _ _] -> _
      timeout: u32 60 ("milliseconds to wait") -> [_ _ _ _ _ _ _ _ _ _ _ _ _ _ _ _ _ _ _ _ _]
      tunnel: w203 -> [w216 _ _ _ _ _ _ _ _ _ _ _ _ _ _ _ _ _ _ _ _]
      tunnel: "Test Tree" -> [_ _ _ _ _ _ _ _ _ _ _ w427 w435 w437 w441 w449 _ _ _ _ _]
      tunnel: w202 -> [_ _ _ _ _ _ _ _ _ _ _ _ _ _ _ _ w462 _ w480 _ _]
      tunnel: w200 -> [_ _ _ _ _ _ _ _ _ _ _ _ _ _ _ _ w458 _ _ _ _]
      tunnel: w199 -> [_ _ _ _ _ _ _ _ _ _ _ _ _ _ _ _ w454 _ _ _ _]
      tunnel: w198 -> [w211 _ _ _ _ _ w378 _ _ _ _ _ _ _ _ _ _ _ _ _ _]
      tunnel: [w210 w255 w357 w362 w371 w375 w376 w385 w395 w402 w414 w426 w433 w436 w440 w448 w453 w475 w477 w481 w492] -> w197
      tunnel: w196 -> [w210 w255 w357 w362 w371 w375 w376 _ _ w402 w414 w426 w433 w436 w440 w448 w453 w475 w477 w481 w492]
      tunnel: w195 -> [w208 _ _ _ _ _ _ _ _ _ _ _ _ _ _ _ _ _ _ _ _]
      event Timeout {
        n110 = event-data() -> ()  [unwired: 1 in, 1 out]
        n111 = local read "Mode"() -> (w213:T4)
        n112 = case shown="\"Basic\"" "Dashboard Tab" {
          tunnel: w216 -> [_ _ w232 _ _]
          tunnel: "/TestMode/Automatic/" ("Name Pattern") -> [_ _ w231 _ _]
          tunnel: T18 [{"Operation"=enum."Clear", "Color Box"=14013909}, {"Operation"=enum."Clear", "Color Box"=14013909}, {"Operation"=enum."Clear", "Color Box"=14013909}, {"Operation"=enum."Clear", "Color Box"=14013909}, {"Operation"=enum."Update", "Color Box"=14013909}, {"Operation"=enum."Update", "Color Box"=16777215}, {"Operation"=enum."Clear", "Color Box"=14013909}, {"Operation"=enum."Clear", "Color Box"=14013909}, {"Operation"=enum."Clear", "Color Box"=14013909}] -> [_ _ w224 _ w248]
          tunnel: w213 -> [_ _ w223 _ w247]
          tunnel: u32[] [15790320, 15790320, 15790320, 15790320, 16777215, 16777215, 15790320, 15790320, 15790320] -> [_ _ _ _ w253]
          tunnel: w211 -> [_ _ _ _ w241]
          tunnel: w208 -> [_ w218 _ _ _]
          frame "Custom", Default {
          }
          frame "Basic" {
            n113 = call <vilib>:"WPI_DashboardUpdateNames.vi"("Controls on Tab"=w218) -> ()  [unwired: 11 in]
          }
          frame "Test" {
            w230 = -2 ("Active Item:Row Number")
            n114 = Index Array(array=w224, index=w223) -> (element=w225:T21)
            n115 = Unbundle(w225) -> ("Operation"=w226:enum16{"Update", "Clear"}, "Color Box"=w227:u32)
            n116 = call <vilib>:"NT Read String.vi"("Name"="/TestMode/TestName") -> ("String"=w221:string)  [unwired: 9 in, 1 out]
            n117 = call <vilib>:"NT Read and Format Entries as Tree.vi"("Operation"=w226, "Name Pattern"=w231, "Tree Refnum"=w232) -> ()  [unwired: 7 in, 2 out]
            n118 = case shown="\"\"" w221 {
              tunnel: "/TestMode/TestProgress" ("Name") -> [w234 _]
              tunnel: "/TestMode/TestProgressText" ("Name") -> [w233 _]
              frame Default {
                n119 = call <vilib>:"NT Read Number.vi"("Name"=w234) -> ("Numeric"=w235:dbl)  [unwired: 9 in, 1 out]
                n120 = call <vilib>:"NT Read String.vi"("Name"=w233) -> ("String"=w236:string)  [unwired: 9 in, 1 out]
                n121 = Bundle("Numeric"=w235, "String"=w236) -> (→"Progress":cluster{"Numeric":dbl, "String":string})  [unwired: 1 in]
              }
              frame "" {
                n122 = property on="Progress" class="Clust (strict)"("Visible"=FALSE) -> ()  [unwired: 2 in, 2 out]
                n123 = local write "Test Name"(u16 0) -> ()
              }
            }
            n124 = property on="Test Tree" class="Tree (strict)"("Active Item Row Number"=w230, "ActiveColNum"=w230, "CellBG"=w227, "Active Item Row Number"=-1 ("Active Item:Row Number"), "CellBG"=u32 5789784 ("Color Box")) -> ()  [unwired: 2 in, 2 out]
          }
          frame "Variables" {
            n125 = control-ref of="Tree"() -> (w240:refnum<vi>)
            n126 = call <vilib>:"NT Read and Format Entries as Tree.vi"("Tree Refnum"=w240) -> ()  [unwired: 9 in, 2 out]
          }
          frame "Commands" {
            w249 = u32 5789784 ("Color Box")
            w250 = T22 {"Row"=-1, "Column"=-2} ("Active Cell:Active Cell")
            w252 = T22 {"Row"=-2, "Column"=-2} ("Active Cell:Active Cell")
            n127 = Index Array(array=w253, index=w247) -> (element=w251:u32)
            n128 = Index Array(array=w248, index=w247) -> (element=w246:T21)
            n129 = Unbundle(w246) -> ("Operation"=w245:enum16{"Update", "Clear"})  [unwired: 1 out]
            n130 = local read "Command Selection"() -> (w244:i32)
            n131 = property on="Command Selection" class="MCListbox (strict)"("ActiveCell"=w252, "CellBG"=w251, "ActiveCell"=w250, "CellBG"=w249) -> ()  [unwired: 2 in, 2 out]
            n132 = call <vilib>:"WPI_DashboardUpdate RPC Info.vi"("Operation"=w245) -> ("update"=w243:bool, "commands"=w242:string[][])  [unwired: 9 in]
            n133 = property on="Command Selection" class="MCListbox (strict)"("ItemNames"=w242) -> ()  [unwired: 2 in, 2 out]
            n134 = property on="Command Params" class="Tbl (strict)"("Active Cell"=w252, "Cell BG Color"=w251, "Active Cell"=w250, "Cell BG Color"=w249) -> ()  [unwired: 2 in, 2 out]
            n135 = call <vilib>:"WPI_DashboardUpdate Command Params.vi"("Update"=w243, "NewVal"=w244, "Commands"=w242, "Param Tbl"=w241) -> ()  [unwired: 7 in, 1 out]
          }
        }
        n136 = call <vilib>:"Connextion Info.vi"() -> ("Connected"=→"NT Connection":bool)  [unwired: 10 in, 1 out]
      }
      event "Test Tree": Value Change {
        # "Show appropriate\ncontrols"
        n137 = event-data() -> ("CtlRef"=w258:refnum<vi>, "NewVal"=w256:string)  [unwired: 1 in]
        n138 = call <vilib>:"WPI_UtilitiesGetTreeIOName.vi"("NewVal"=w256, "TreeControl in"=w258) -> ("I/O Name"=w259:string)  [unwired: 9 in]
        n139 = case shown="\"Camera\"" w259 {
          selector: w259 -> [_ w266 _ w288 w297 _]
          tunnel: w256 -> [_ _ w285 w287 _ w304]
          tunnel: cluster{string[]}[] [{["640x480", "320x240", "160x120"]}, {["Auto", "Fixed indoor", "Fixed outdoor 1", "Fixed outdoor 2", "Fixed fluorescent 1", "Fixed fluorescent 2", "Hold current"]}, {["Auto", "Flicker-free 50 Hz", "Flicker-free 60 Hz", "Hold current"]}, {["None", "Prioritize frame rate", "Prioritize image quality"]}, {["Monochrome", "Color"]}] -> [_ _ _ _ _ w303]
          frame Default {
            w261 = FALSE ("Visible")
            w260 = FALSE ("Visible")
            n140 = property on="Motor" class="Clust (strict)"("Visible"=w260) -> ()  [unwired: 2 in, 2 out]
            n141 = property on="Test Ring" class="Ring (strict)"("Visible"=w260) -> ()  [unwired: 2 in, 2 out]
            n142 = property on="Rev/Fwd" class="Clust (strict)"("Visible"=w261) -> ()  [unwired: 2 in, 2 out]
            n143 = property on="On/Off" class="Bool (strict)"("Visible"=w261) -> ()  [unwired: 2 in, 2 out]
            n144 = property on="Test Slider" class="Slide (strict)"("Visible"=w261) -> ()  [unwired: 2 in, 2 out]
          }
          frame "Analog Out", "Motor", "PWM" {
            w267 = FALSE ("Visible")
            n145 = case shown="\"Analog Out\"" w266 {
              tunnel: [1.0 ("Value") -1.0 ("Value") 0.0 ("Value")] -> w265
              tunnel: [255.0 ("Value") 1.0 ("Value") 5.0 ("Value")] -> w264
              tunnel: [128.0 ("Value") 0.0 ("Value") 0.0 ("Value")] -> w263
              tunnel: [64.0 ("Value") 0.5 ("Value") 1.0 ("Value")] -> w262
              frame "PWM" {
              }
              frame "Motor", Default {
              }
              frame "Analog Out" {
              }
            }
            n146 = property on="Motor" class="Clust (strict)"("Visible"=TRUE) -> ()  [unwired: 2 in, 2 out]
            n147 = property on="Value" class="Slide (strict)"("Value"=w263, "Scale.Minimum"=w265, "Scale.Maximum"=w264, "Scale.Increment"=w262) -> ()  [unwired: 2 in, 2 out]
            n148 = property on="On/Off" class="Bool (strict)"("Visible"=w267) -> ()  [unwired: 2 in, 2 out]
            n149 = property on="Test Slider" class="Slide (strict)"("Visible"=w267) -> ()  [unwired: 2 in, 2 out]
            n150 = property on="Test Ring" class="Ring (strict)"("Visible"=w267) -> ()  [unwired: 2 in, 2 out]
            n151 = property on="Rev/Fwd" class="Clust (strict)"("Visible"=w267) -> ()  [unwired: 2 in, 2 out]
          }
          frame "Servo" {
            w283 = FALSE ("Visible")
            n152 = call <vilib>:"NT Read Number.vi"("Name"=w285) -> ("Numeric"=w284:dbl)  [unwired: 9 in, 1 out]
            n153 = property on="Test Slider" class="Slide (strict)"("Visible"=TRUE, "Scale.Maximum"=170.0 ("Scale.Range:Maximum")) -> ()  [unwired: 2 in, 2 out]
            n154 = local write "Test Slider"(w284) -> ()
            n155 = property on="Motor" class="Clust (strict)"("Visible"=w283) -> ()  [unwired: 2 in, 2 out]
            n156 = property on="Rev/Fwd" class="Clust (strict)"("Visible"=w283) -> ()  [unwired: 2 in, 2 out]
            n157 = property on="On/Off" class="Bool (strict)"("Visible"=w283) -> ()  [unwired: 2 in, 2 out]
            n158 = property on="Test Ring" class="Ring (strict)"("Visible"=w283) -> ()  [unwired: 2 in, 2 out]
          }
          frame "Relay", "Solenoid" {
            w286 = FALSE ("Visible")
            n159 = property on="Motor" class="Clust (strict)"("Visible"=w286) -> ()  [unwired: 2 in, 2 out]
            n160 = property on="Test Slider" class="Slide (strict)"("Visible"=w286) -> ()  [unwired: 2 in, 2 out]
            n161 = Search and Replace String(input string=w287, search string="/Value  **", replace string="/Direction") -> (result string=w293:string)  [unwired: 5 in, 3 out]
            n162 = property on="Test Ring" class="Ring (strict)"("Visible"=w286) -> ()  [unwired: 2 in, 2 out]
            n163 = call <vilib>:"NT Read String.vi"("Name"=w293) -> ("String"=w291:string)  [unwired: 9 in, 1 out]
            n164 = Equal?(x="Both directions", y=w291) -> (x = y?=w289:bool)
            n165 = Not(x=w289) -> (.not. x?=w290:bool)
            n166 = property on="Rev/Fwd" class="Clust (strict)"("Visible"=w289) -> ()  [unwired: 2 in, 2 out]
            n167 = property on="On/Off" class="Bool (strict)"("Visible"=w290, "Caption.Text"=w288) -> ()  [unwired: 2 in, 2 out]
          }
          frame "Compressor", "Digital Out" {
            w296 = FALSE ("Visible")
            # "Get direction and finish"
            n168 = property on="Motor" class="Clust (strict)"("Visible"=w296) -> ()  [unwired: 2 in, 2 out]
            n169 = property on="Test Slider" class="Slide (strict)"("Visible"=w296) -> ()  [unwired: 2 in, 2 out]
            n170 = property on="Test Ring" class="Ring (strict)"("Visible"=w296) -> ()  [unwired: 2 in, 2 out]
            n171 = property on="On/Off" class="Bool (strict)"("Visible"=TRUE, "Caption.Text"=w297) -> ()  [unwired: 2 in, 2 out]
            n172 = property on="Rev/Fwd" class="Clust (strict)"("Visible"=FALSE) -> ()  [unwired: 2 in, 2 out]
          }
          frame "Camera" {
            n173 = call <vilib>:"Get Last Path Segment.vi"("String in"=w304) -> ("String out"=w305:string)  [unwired: 10 in]
            n174 = property on="On/Off" class="Bool (strict)"("Visible"=FALSE) -> ()  [unwired: 2 in, 2 out]
            n175 = property on="Motor" class="Clust (strict)"("Visible"=FALSE) -> ()  [unwired: 2 in, 2 out]
            n176 = property on="Rev/Fwd" class="Clust (strict)"("Visible"=FALSE) -> ()  [unwired: 2 in, 2 out]
            n177 = case shown="\"White Balance  **\"" w305 {
              tunnel: w304 -> [w311 w320 w329 w338 w347 _ w353]
              tunnel: w303 -> [w309 w317 w326 w335 w344 _ _]
              frame "Size  **" {
                n178 = Index Array(array=w309) -> (element=w308:cluster{string[]})  [unwired: 1 in]
                n179 = call <vilib>:"NT Read String.vi"("Name"=w311) -> ("String"=w310:string)  [unwired: 9 in, 1 out]
                n180 = Unbundle(w308) -> (w306:string[])
                n181 = Match First String(2:w306, 3:w310) -> (0:w307:i32)  [unwired: 1 out]
                n182 = property on="Test Ring" class="Ring (strict)"("Value"=w307, "Strings []"=w306) -> ()  [unwired: 2 in, 2 out]
                n183 = property on="Test Ring" class="Ring (strict)"("Visible"=TRUE) -> ()  [unwired: 2 in, 2 out]
                n184 = property on="Test Slider" class="Slide (strict)"("Visible"=FALSE) -> ()  [unwired: 2 in, 2 out]
              }
              frame "White Balance  **" {
                n185 = Index Array(array=w317, index=1) -> (element=w318:cluster{string[]})
                n186 = call <vilib>:"NT Read String.vi"("Name"=w320) -> ("String"=w319:string)  [unwired: 9 in, 1 out]
                n187 = Unbundle(w318) -> (w315:string[])
                n188 = Match First String(2:w315, 3:w319) -> (0:w314:i32)  [unwired: 1 out]
                n189 = property on="Test Ring" class="Ring (strict)"("Value"=w314, "Strings []"=w315) -> ()  [unwired: 2 in, 2 out]
                n190 = property on="Test Ring" class="Ring (strict)"("Visible"=TRUE) -> ()  [unwired: 2 in, 2 out]
                n191 = property on="Test Slider" class="Slide (strict)"("Visible"=FALSE) -> ()  [unwired: 2 in, 2 out]
              }
              frame "Exposure  **" {
                n192 = Index Array(array=w326, index=2) -> (element=w327:cluster{string[]})
                n193 = call <vilib>:"NT Read String.vi"("Name"=w329) -> ("String"=w328:string)  [unwired: 9 in, 1 out]
                n194 = Unbundle(w327) -> (w323:string[])
                n195 = Match First String(2:w323, 3:w328) -> (0:w324:i32)  [unwired: 1 out]
                n196 = property on="Test Ring" class="Ring (strict)"("Value"=w324, "Strings []"=w323) -> ()  [unwired: 2 in, 2 out]
                n197 = property on="Test Ring" class="Ring (strict)"("Visible"=TRUE) -> ()  [unwired: 2 in, 2 out]
                n198 = property on="Test Slider" class="Slide (strict)"("Visible"=FALSE) -> ()  [unwired: 2 in, 2 out]
              }
              frame "Exposure Priority  **" {
                n199 = Index Array(array=w335, index=3) -> (element=w336:cluster{string[]})
                n200 = call <vilib>:"NT Read String.vi"("Name"=w338) -> ("String"=w337:string)  [unwired: 9 in, 1 out]
                n201 = Unbundle(w336) -> (w332:string[])
                n202 = Match First String(2:w332, 3:w337) -> (0:w333:i32)  [unwired: 1 out]
                n203 = property on="Test Ring" class="Ring (strict)"("Value"=w333, "Strings []"=w332) -> ()  [unwired: 2 in, 2 out]
                n204 = property on="Test Ring" class="Ring (strict)"("Visible"=TRUE) -> ()  [unwired: 2 in, 2 out]
                n205 = property on="Test Slider" class="Slide (strict)"("Visible"=FALSE) -> ()  [unwired: 2 in, 2 out]
              }
              frame "Color Enable  **" {
                n206 = Index Array(array=w344, index=4) -> (element=w345:cluster{string[]})
                n207 = call <vilib>:"NT Read String.vi"("Name"=w347) -> ("String"=w346:string)  [unwired: 9 in, 1 out]
                n208 = Unbundle(w345) -> (w341:string[])
                n209 = Match First String(2:w341, 3:w346) -> (0:w342:i32)  [unwired: 1 out]
                n210 = property on="Test Ring" class="Ring (strict)"("Value"=w342, "Strings []"=w341) -> ()  [unwired: 2 in, 2 out]
                n211 = property on="Test Ring" class="Ring (strict)"("Visible"=TRUE) -> ()  [unwired: 2 in, 2 out]
                n212 = property on="Test Slider" class="Slide (strict)"("Visible"=FALSE) -> ()  [unwired: 2 in, 2 out]
              }
              frame Default {
                n213 = property on="Test Ring" class="Ring (strict)"("Visible"=FALSE) -> ()  [unwired: 2 in, 2 out]
                n214 = property on="Test Slider" class="Slide (strict)"("Visible"=FALSE) -> ()  [unwired: 2 in, 2 out]
              }
              frame "Brightness  **", "Color Level  **", "Compression  **", "FPS  **", "Sharpness  **" {
                n215 = call <vilib>:"NT Read Number.vi"("Name"=w353) -> ("Numeric"=w352:dbl)  [unwired: 9 in, 1 out]
                n216 = local write "Test Slider"(w352) -> ()
                n217 = property on="Test Slider" class="Slide (strict)"("Visible"=TRUE, "Scale.Maximum"=100.0 ("Scale.Range:Maximum")) -> ()  [unwired: 2 in, 2 out]
                n218 = property on="Test Ring" class="Ring (strict)"("Visible"=FALSE) -> ()  [unwired: 2 in, 2 out]
              }
            }
          }
        }
        n219 = property on="Progress" class="Clust (strict)"("Visible"=FALSE) -> ()  [unwired: 2 in, 2 out]
      }
      event "Test Name": Mouse Enter {
        # "Populate the ring with the list of tests"
        n220 = event-data() -> ()  [unwired: 1 in, 1 out]
        n221 = call <vilib>:"NT Read String Array.vi"("Name"="/TestMode/TestList") -> ("String Array"=w361:string[])  [unwired: 9 in, 1 out]
        n222 = Build Array (concatenate)("Select the test to run...", w361) -> (w360:string[])
        n223 = property on="Test Name" class="Ring (strict)"("Strings []"=w360) -> ()  [unwired: 2 in, 2 out]
      }
      event "Test Name": Value Change {
        w363 = FALSE ("Visible")
        # "Tell the robot the test name to run"
        n224 = event-data() -> ("NewVal"=w367:u16)  [unwired: 1 in]
        n225 = property on="Test Name" class="Ring (strict)"() -> ("Strings []"=w368:string[])  [unwired: 2 in, 2 out]
        n226 = local write "Progress"(T6 {"Test Progress"=0, "Test Progress Text"=""} ("Progress")) -> ()
        n227 = Index Array(array=w368, index=w367) -> (element=w366:string)
        n228 = call <vilib>:"NT Write String.vi"("String"=w366, "Name"="/TestMode/TestName") -> ()  [unwired: 9 in, 1 out]
        n229 = property on="Progress" class="Clust (strict)"("Visible"=TRUE) -> ()  [unwired: 2 in, 2 out]
        n230 = property on="Motor" class="Clust (strict)"("Visible"=w363) -> ()  [unwired: 2 in, 2 out]
        n231 = property on="Test Slider" class="Slide (strict)"("Visible"=w363) -> ()  [unwired: 2 in, 2 out]
        n232 = property on="On/Off" class="Bool (strict)"("Visible"=w363) -> ()  [unwired: 2 in, 2 out]
        n233 = property on="Rev/Fwd" class="Clust (strict)"("Visible"=w363) -> ()  [unwired: 2 in, 2 out]
        n234 = property on="Test Ring" class="Ring (strict)"("Visible"=w363) -> ()  [unwired: 2 in, 2 out]
      }
      event "Select Auto": Mouse Enter {
        # "Populate the combo box with the list of autonomous options"
        n235 = event-data() -> ()  [unwired: 1 in, 1 out]
        n236 = call <vilib>:"NT Read String Array.vi"("Name"="Auto List") -> ("String Array"=w370:string[])  [unwired: 9 in, 1 out]
        n237 = property on="Select Auto" class="CmbBox"("Strings[]"=w370) -> ()  [unwired: 2 in, 2 out]
      }
      event "Select Auto": Value Change {
        # "User modified the Auto Selection. Write to NT variable so robot knows."
        n238 = event-data() -> ("NewVal"=w373:string)  [unwired: 1 in]
        n239 = call <vilib>:"NT Write String.vi"("String"=w373, "Name"="Auto Selector") -> ()  [unwired: 9 in, 1 out]
      }
      event "Command Selection": Value Change {
        # "Get the params and show in table"
        n240 = event-data() -> ("NewVal"=w379:i32)  [unwired: 1 in]
        n241 = property on="Command Selection" class="MCListbox (strict)"() -> ("ItemNames"=w377:string[][])  [unwired: 2 in, 2 out]
        n242 = call <vilib>:"WPI_DashboardUpdate Command Params.vi"("NewVal"=w379, "Commands"=w377, "Param Tbl"=w378) -> ()  [unwired: 8 in, 1 out]
      }
      event "Execute Command": Value Change {
        # "Started one, Unique ID holds\nresponse"
        n243 = event-data() -> ()  [unwired: 1 in, 1 out]
        n244 = property on="Command Selection" class="MCListbox (strict)"() -> ("ItemNames"=w390:string[][])  [unwired: 2 in, 2 out]
        n245 = Index Array(array=w390, index (row)="Command Selection", index (col)=0) -> (element=w388:string)
        n246 = call <vilib>:"Invoke Commands.vi"("Command Params"="Command Params", "Function Name"=w388) -> ("Params"=w384:u8, "Started"=w383:bool)  [unwired: 7 in, 1 out]
        n247 = Array Subset(array="Command Params", length (row)=w384) -> (w385:string[][])  [unwired: 3 in]
        n248 = Select(t="Executing" ("Cmd Status"), s=w383, f="" ("Cmd Status")) -> (s? t:f=→"Cmd Status":string)
      }
      event "Command Selection": Double Click {
        n249 = event-data() -> ("Row"=w398:i32)  [unwired: 1 in]
        n250 = property on="Command Selection" class="MCListbox (strict)"() -> ("ItemNames"=w401:string[][])  [unwired: 2 in, 2 out]
        n251 = local read "Command Params"() -> (w397:string[][])
        n252 = Index Array(array=w401, index (row)=w398, index (col)=0) -> (element=w399:string)
        n253 = call <vilib>:"Invoke Commands.vi"("Command Params"=w397, "Function Name"=w399) -> ("Params"=w396:u8, "Started"=w391:bool)  [unwired: 7 in, 1 out]
        n254 = Array Subset(array=w397, length (row)=w396) -> (w395:string[][])  [unwired: 3 in]
        n255 = Select(t="Executing" ("Cmd Status"), s=w391, f="" ("Cmd Status")) -> (s? t:f=w392:string)
        n256 = local write "Cmd Status"(w392) -> ()
      }
      event "CheckList": Double Click {
        # "Shift clears all"
        # "Update symbols on the listbox"
        n257 = event-data() -> ("PlatMods.Shift"=w403:bool, "Row"=w405:i32)  [unwired: 1 in]
        n258 = case shown="True" w403 {
          tunnel: w405 -> [w409 _]
          tunnel: 1 -> [w408 _]
          frame False {
            n259 = property on="CheckList" class="LstBox (strict)"() -> ("Item Symbols"=w407:i32[])  [unwired: 2 in, 2 out]
            n260 = Replace Array Subset(array=w407, new element=w408, index=w409) -> (w406:i32[])
            n261 = property on="CheckList" class="LstBox (strict)"("Item Symbols"=w406) -> ()  [unwired: 2 in, 2 out]
          }
          frame True {
            w410 = 0 ("Top Row")
            n262 = property on="CheckList" class="LstBox (strict)"() -> ("Number of Rows"=w412:u32)  [unwired: 2 in, 2 out]
            n263 = Initialize Array(0, w412) -> (w411:i32[])
            n264 = property on="CheckList" class="LstBox (strict)"("Top Row"=w410, "Value"=w410, "Item Symbols"=w411) -> ()  [unwired: 2 in, 2 out]
          }
        }
      }
      event "CheckList": Key Down {
        # "Update symbols on the listbox\nLeft and right keys check and uncheck"
        n265 = event-data() -> ("VKey"=w416:T19)  [unwired: 1 in]
        n266 = case shown="\"Left\", \"Right\"" w416 {
          selector: w416 -> [w421 _]
          tunnel: eventvkey."Left" ("VKey") -> [w419 _]
          frame "Left", "Right" {
            n267 = Equal?(x=w419, y=w421) -> (x = y?=w420:bool)
            n268 = Select(t=0, s=w420, f=1) -> (s? t:f=w422:i32)
            n269 = property on="CheckList" class="LstBox (strict)"() -> ("Item Symbols"=w425:i32[])  [unwired: 2 in, 2 out]
            n270 = Replace Array Subset(array=w425, new element=w422, index="CheckList") -> (w424:i32[])
            n271 = property on="CheckList" class="LstBox (strict)"("Item Symbols"=w424) -> ()  [unwired: 2 in, 2 out]
          }
          frame Default {
          }
        }
      }
      event "Motor.Enable": Value Change {
        # "When the test mode otor enable helper is set, update that\ntree row item's value"
        n272 = event-data() -> ("NewVal"=w431:bool)  [unwired: 1 in]
        n273 = Unbundle("Motor") -> ("Value"=w430:dbl)  [unwired: 1 out]
        n274 = Select(t=w430, s=w431, f=0.0) -> (s? t:f=w428:dbl)
        n275 = call <vilib>:"NT Write Number.vi"("Numeric"=w428, "Name"=w427) -> ()  [unwired: 9 in, 1 out]
      }
      event "Test Slider": Value Change {
        # "When the test mode slider helper is set, update that\ntree row item's value"
        n276 = event-data() -> ("NewVal"=w434:dbl)  [unwired: 1 in]
        n277 = call <vilib>:"NT Write Number.vi"("Numeric"=w434, "Name"=w435) -> ()  [unwired: 9 in, 1 out]
      }
      event "On/Off": Value Change {
        # "When the test mode on/off helper value is set, update that\ntree row item's value"
        n278 = event-data() -> ("NewVal"=w439:bool)  [unwired: 1 in]
        n279 = Boolean To (0,1)(Boolean=w439) -> (0, 1=w438:i16)
        n280 = call <vilib>:"NT Write Number.vi"("Numeric"=w438, "Name"=w437) -> ()  [unwired: 9 in, 1 out]
      }
      event "Rev/Fwd": Value Change {
        # "When the test mode helper value for relays is set, update that\ntree row item's value"
        n281 = event-data() -> ("NewVal.Forward"=w447:bool, "NewVal.Reverse"=w446:bool)  [unwired: 1 in]
        n282 = Boolean To (0,1)(Boolean=w447) -> (0, 1=w443:i16)
        n283 = Boolean To (0,1)(Boolean=w446) -> (0, 1=w445:i16)
        n284 = Negate(x=w445) -> (-x=w444:i16)
        n285 = Add(x=w443, y=w444) -> (x+y=w442:i16)
        n286 = call <vilib>:"NT Write Number.vi"("Numeric"=w442, "Name"=w441) -> ()  [unwired: 9 in, 1 out]
      }
      event "Test Ring": Value Change {
        # "When a test mode helper value is selected from the ring,\nset the tree item's variable to the string value"
        n287 = event-data() -> ("NewVal"=w451:u16)  [unwired: 1 in]
        n288 = property on="Test Ring" class="Ring (strict)"() -> ("Strings []"=w452:string[])  [unwired: 2 in, 2 out]
        n289 = Index Array(array=w452, index=w451) -> (element=w450:string)
        n290 = call <vilib>:"NT Write String.vi"("String"=w450, "Name"=w449) -> ()  [unwired: 9 in, 1 out]
      }
      event "Rec Mode": Value Change {
        # "Update globals for recording mode and path to read log from.\nClear when logging and let NetworkTables set path for vision to\nuse."
        n291 = event-data() -> ("NewVal"=w463:enum32{"Stop", "Record", "Playback"})  [unwired: 1 in]
        n292 = global write "WPI_DashboardLogging Global.vi" "Logging Filename"(path "") -> ()
        n293 = global write "WPI_DashboardLogging Global.vi" "Recording"(w463) -> ()
        n294 = case shown="\"Playback\"" w463 {
          tunnel: w462 -> [_ w465 w474]
          tunnel: [_ _ w473] -> w460
          tunnel: [_ _ w472] -> _
          tunnel: w458 -> [_ _ w470]
          tunnel: cluster{i32, i32} {-250, 170} -> [_ _ w469]
          tunnel: [_ _ T20 {"Image Size"=TRUE, "Image Type"=TRUE, "Pixel Value"=TRUE, "ROI Information"=TRUE, "Zoom Factor"=FALSE} ("Image Information Shown:All Elements")] -> w456
          tunnel: [_ _ TRUE ("Zoom Factor")] -> w455
          tunnel: w454 -> [_ _ w466]
          frame Default {
          }
          frame "Stop", "Record" {
            # "Place Window too"
            n295 = invoke class="VI" method="FP.Close"(reference=w465) -> (reference out=w464:refnum<vi>)  [unwired: 2 in, 2 out]
            n296 = invoke class="VI" method="Abort VI"(reference=w464) -> ()  [unwired: 2 in, 3 out]
          }
          frame "Playback" {
            n297 = call "Open Playback Panel.vi"("Offset"=w469, "DB VI Ref"=w470, "Playback in"=w474) -> ("Playback out"=w471:refnum<vi>)  [unwired: 8 in]
            n298 = register-events(w471, w466) -> (reference out=w473:refnum<event-registration>, error out=w472:errorcluster)  [unwired: 2 in]
          }
        }
        n299 = property on="Camera Image" class="ImageControl"("Image Information Shown"=w456, "Image Information Visible"=w455) -> ()  [unwired: 2 in, 2 out]
        n300 = call <vilib>:"WPI_DashboardNT Log FieldName Cache.vi"("Operation"=enum16{"Lookup/Add", "Index", "Clear"}."Clear") -> ()  [unwired: 8 in, 3 out]
      }
      event Panel Close {
        w476 = enum32{"Stop", "Record", "Playback"}."Stop" ("Rec Mode")
        # "Playback window has been closed, abort"
        n301 = event-data() -> ()  [unwired: 1 in, 4 out]
        n302 = local write "Rec Mode"(w476) -> ()
        n303 = global write "WPI_DashboardLogging Global.vi" "Recording"(w476) -> ()
      }
      event Panel Close {
        # "Abort playback window and ourself"
        n304 = event-data() -> ()  [unwired: 1 in, 4 out]
        n305 = invoke class="VI" method="FP.Close"(reference=w480) -> (reference out=w479:refnum<vi>)  [unwired: 2 in, 2 out]
        n306 = invoke class="VI" method="Abort VI"(reference=w479) -> (error out=w478:errorcluster)  [unwired: 2 in, 2 out]
        n307 = invoke class="VI" method="Abort VI"(error in=w478) -> ()  [unwired: 2 in, 3 out]
      }
      event User Event {
        n308 = event-data() -> ("IDs"=w487:cluster{"RPC field ID":u16, "Unique ID":u16}, "String"=w486:string)  [unwired: 1 in]
        n309 = Bundle("IDs"=w487, "String"=w486) -> (w485:T8)  [unwired: 1 in]
        n310 = call <vilib>:"Retrieve RPC Response.vi"("RPC Response"=w485) -> ("Output"=w483:string[][])  [unwired: 10 in]
        n311 = Build Array (concatenate)(w481, w483) -> (w482:string[][])
        n312 = local write "Command Params"(w482) -> ()
        n313 = local write "Cmd Status"("" ("Cmd Status")) -> ()
      }
      event "Tree": Double Click {
        n314 = event-data() -> ("PlatMods"=w491:T23, "Tag"=w490:string)  [unwired: 1 in]
        n315 = Unbundle(w491) -> ("Shift"=w489:bool)  [unwired: 4 out]
        n316 = Not(x=w489) -> (.not. x?=w488:bool)
        n317 = call <vilib>:"NT Update Persistence.vi"("Persistence"=w488, "Name"=w490) -> ()  [unwired: 9 in, 1 out]
      }
    }
  }
  n318 = while {
    tunnel: w64 -> [w494]
    i -> [w497]
    stop <- FALSE stop-if-true
    n319 = Wait (ms)(milliseconds to wait=u32 100) -> ()  [unwired: 1 out]
    n320 = case shown="\"Playback\"" "Rec Mode" {
      tunnel: w497 -> [_ _ w512]
      tunnel: [u32 2829099 ("Base Color") u32 11141120 ("Target Color") w501] -> w493
      frame "Stop", Default {
        # "Reset the color, extra updates don't cost much"
      }
      frame "Record" {
      }
      frame "Playback" {
        # "Playback"
        n321 = Quotient & Remainder(x=w512, y=u32 50 ("milliseconds to wait")) -> (x-y*floor(x/y)=w508:u32)  [unwired: 1 out]
        n322 = Divide(x=w508, y=u32 50 ("milliseconds to wait")) -> (x/y=w505:dbl)
        n323 = Multiply(x=6.283185307179586, y=w505) -> (x*y=w510:dbl)
        n324 = Sine(x=w510) -> (sin(x)=w509:dbl)
        n325 = Absolute Value(x=w509) -> (abs(x)=w502:dbl)
        n326 = call "Interpolate RGB Color.vi"("Proportion"=w502, "Target Color"=u32 30976, "Base Color"=u32 2829099) -> ("Result Color"=w501:u32)  [unwired: 8 in]
      }
    }
    n327 = property class="Pane"(reference=w494, "PaneColor"=w493) -> ()  [unwired: 1 in, 2 out]
  }
  n328 = local write "Dashboard Tab"(T2."Drive" ("Dashboard Tab")) -> ()
  n329 = property on="On/Off" class="Bool (strict)"("Visible"=w33) -> ()  [unwired: 2 in, 2 out]
  n330 = property on="Motor" class="Clust (strict)"("Visible"=w33) -> ()  [unwired: 2 in, 2 out]
  n331 = property on="Progress" class="Clust (strict)"("Visible"=w33) -> ()  [unwired: 2 in, 2 out]
  n332 = property on="Test Ring" class="Ring (strict)"("Visible"=w33) -> ()  [unwired: 2 in, 2 out]
  n333 = property on="Rev/Fwd" class="Clust (strict)"("Visible"=w33) -> ()  [unwired: 2 in, 2 out]
  n334 = while {
    tunnel: u16 1741 ("timeout ms (25000)") -> [w514]
    stop <- FALSE stop-if-true
    n335 = TCP Create Listener(10:w514) -> (0:w513:errorcluster, 3:w515:refnum<k5>)  [unwired: 4 in, 1 out]
    n336 = case shown="No Error" w513 {
      selector: w513 -> [w517 _]
      tunnel: w515 -> [w518 _]
      frame No Error {
        n337 = while {
          tunnel: w518 -> [w521]
          tunnel: w517 -> [w520]
          stop <- FALSE stop-if-true
          n338 = TCP Wait On Listener(8:w520, 11:w521) -> (0:w522:errorcluster, 4:w523:refnum<k5>)  [unwired: 2 in, 3 out]
          n339 = local write "TCP"(w523) -> ()
          n340 = case shown="No Error" w522 {
            frame No Error {
            }
            frame Error {
              n341 = Wait (ms)(milliseconds to wait=u32 1000) -> ()  [unwired: 1 out]
            }
          }
        }
      }
      frame Error {
        n342 = Wait (ms)(milliseconds to wait=u32 1000) -> ()  [unwired: 1 out]
      }
    }
  }
  n343 = local write "Command Selection"(u16 0 ("milliseconds to wait")) -> ()
  n344 = local write "Command Params"(string[][] [] ("Command Params")) -> ()
  n345 = global write "WPI_DashboardLogging Global.vi" "Recording"(w58) -> ()
  n346 = local write "Rec Mode"(w58) -> ()
  n347 = call <vilib>:"NT Write String.vi"("String"="Select Auto", "Name"="Auto Selector") -> ()  [unwired: 9 in, 1 out]
